vi "AlliGator Get IRF Values & Locations.vi"(10 "[IRF Data]":dbl[][](array[numeric])) -> (1 "IRF Locations":cluster{"X":i32, "Y":i32}[](array[cluster]), 2 "[IRF Values]":dbl[][](array[numeric]))   [LabVIEW 2021, in "AlliGator IRF.lvlib"]
doc: "Gets the array of stored <B>IRF Values</B> as well as the <B>IRF Locations</B>."
uses:
  AlliGator IRF.lvlib
panel:
  out "Error Out":errorcluster
  in  "Error In":errorcluster
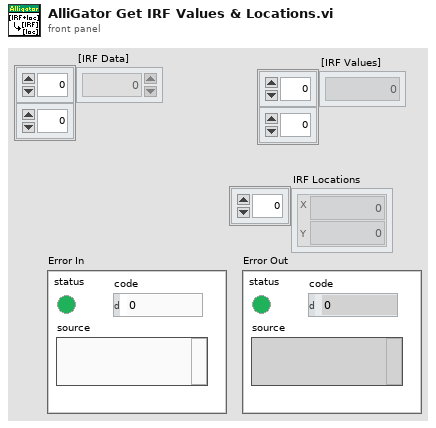
[diagram p1: front panel]
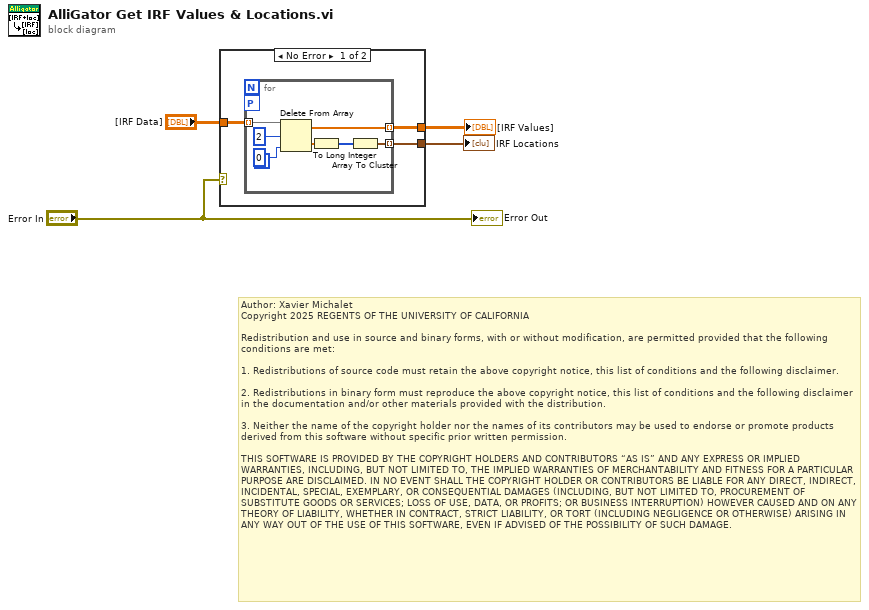
[diagram p0: block diagram]
diagram:
  # "Author: Xavier Michalet\nCopyright 2025 REGENTS OF THE UNIVERSITY OF CALIFORNIA\n\nRedistribution and use in source and binary forms, with or without modification, are permitted provided that the following conditions are met:\n\n1. Redistributions of source code must retain the above copyright notice, this list of conditions and the following disclaimer.\n\n2. Redistributions in binary form must reproduce the above copyright notice, this list of conditions and the following disclaimer in the documentation and/or other materials provided with the distribution.\n\n3. Neither the name of the copyright holder nor the names of its contributors may be used to endorse or promote products derived from this software without specific prior written permission.\n\nTHIS SOFTWARE IS PROVIDED BY THE COPYRIGHT HOLDERS AND CONTRIBUTORS “AS IS” AND ANY EXPRESS OR IMPLIED WARRANTIES, INCLUDING, BUT NOT LIMITED TO, THE IMPLIED WARRANTIES OF MERCHANTABILITY AND FITNESS FOR A PARTICULAR PURPOSE ARE DISCLAIMED. IN NO EVENT SHALL THE COPYRIGHT HOLDER OR CONTRIBUTORS BE LIABLE FOR ANY DIRECT, INDIRECT, INCIDENTAL, SPECIAL, EXEMPLARY, OR CONSEQUENTIAL DAMAGES (INCLUDING, BUT NOT LIMITED TO, PROCUREMENT OF SUBSTITUTE GOODS OR SERVICES; LOSS OF USE, DATA, OR PROFITS; OR BUSINESS INTERRUPTION) HOWEVER CAUSED AND ON ANY THEORY OF LIABILITY, WHETHER IN CONTRACT, STRICT LIABILITY, OR TORT (INCLUDING NEGLIGENCE OR OTHERWISE) ARISING IN ANY WAY OUT OF THE USE OF THIS SOFTWARE, EVEN IF ADVISED OF THE POSSIBILITY OF SUCH DAMAGE."
  n1 = case shown="No Error" "Error In" {
    tunnel: "[IRF Data]" -> [w7 _]
    tunnel: [w6 _] -> w3
    tunnel: [w5 _] -> w2
    frame No Error {
      n2 = for {
        tunnel: w7 -> [w12] mode=indexing
        tunnel: [w11] -> w6 mode=indexing
        tunnel: [w9] -> w5 mode=indexing
        workers-P: _ -> [_]
        n3 = Delete From Array(array=w12, length=2, index=0) -> (deleted portion=w10:dbl[], array with subset deleted=w11:dbl[])
        n4 = To Long Integer(number=w10) -> (32bit integer=w8:i32[])
        n5 = Array To Cluster(array=w8) -> (cluster=w9:cluster{"[0]":i32, "[1]":i32})
      }
    }
    frame Error {
    }
  }
  "[IRF Values]" <- w3
  "IRF Locations" <- w2
  "Error Out" <- "Error In"
